vi "Chart & graph MC.vi"() -> ()   [LabVIEW 2012]
panel:
  out "Waveform Graph":T1(graph)
  in  "Fine":bool
  in  "n° punti":i32=100
  in  "intervallo [s]":sgl=0.1 format="%.2f"
  in  "istante iniz.":dbl format="%.2f"
  in  "STOP":bool
  out "Waveform Chart":dbl(graph)
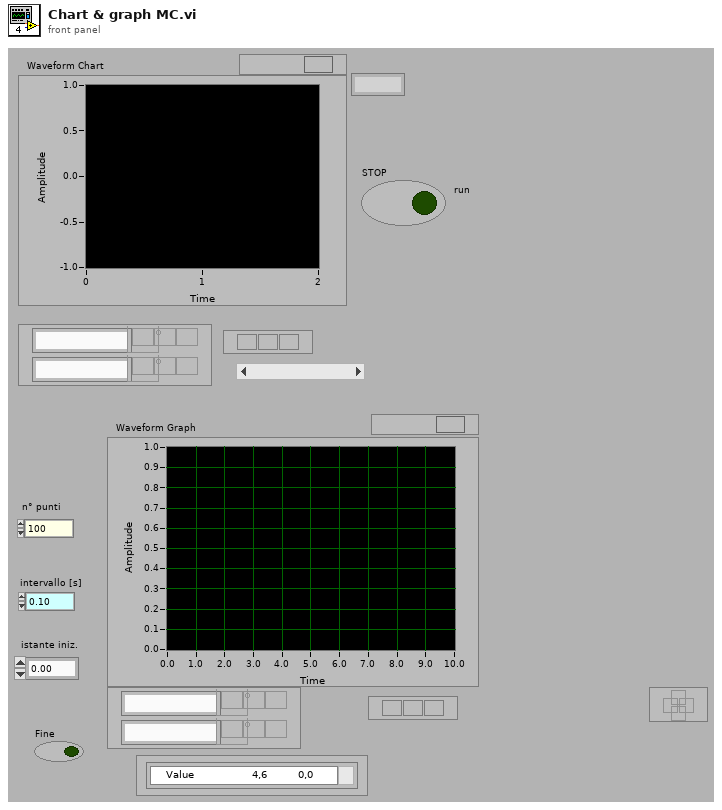
[diagram p1: front panel]
types:
  T1 = cluster{"istante iniz.":dbl, "intervallo [s]":sgl, dbl[][]}
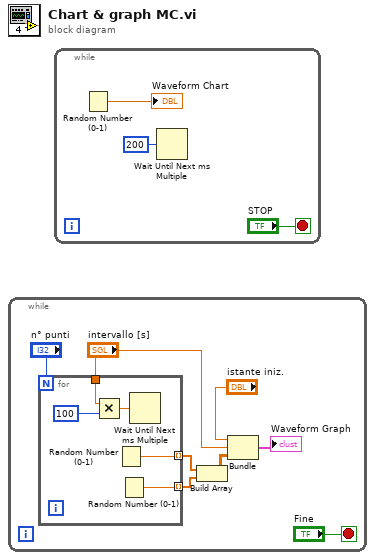
[diagram p0: block diagram]
diagram:
  n1 = while {
    stop <- "Fine" stop-if-true
    n2 = for {
      N: "n° punti" -> [_]
      tunnel: [w13] -> w3 mode=indexing
      tunnel: "intervallo [s]" -> [w11]
      tunnel: [w9] -> w2 mode=indexing
      n3 = Multiply(x=w11, y=100) -> (x*y=w12:sgl)
      n4 = Random Number (0-1)() -> (number: 0 to 1=w13:dbl)
      n5 = Random Number (0-1)() -> (number: 0 to 1=w9:dbl)
      n6 = Wait Until Next ms Multiple(millisecond multiple=w12) -> ()  [unwired: 1 out]
    }
    n7 = Build Array(w3, w2) -> (w1:dbl[][])
    n8 = Bundle("istante iniz."="istante iniz.", "intervallo [s]"="intervallo [s]", w1) -> (→"Waveform Graph":T1)  [unwired: 1 in]
  }
  n9 = while {
    stop <- "STOP" stop-if-true
    n10 = Random Number (0-1)() -> (number: 0 to 1=→"Waveform Chart":dbl)
    n11 = Wait Until Next ms Multiple(millisecond multiple=u32 200) -> ()  [unwired: 1 out]
  }
